vi "Test Program Read Tag Data.vi"(8 "error in (no error)":errorcluster, 10 "Data Cluster":T1, 11 "Task D-O Channels":string[][](array[string])) -> (0 "error out":errorcluster, 3 "Array":bool[][](array[boolean]))   [LabVIEW 2018, in "DAQ.lvlib"]
uses:
  DAQ.lvlib
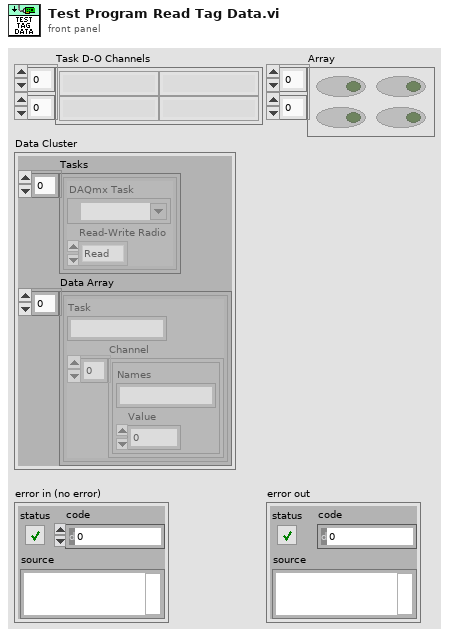
[diagram p1: front panel]
types:
  T1 = cluster{"Tasks":cluster{"DAQmx Task":refnum<k21>, "Read-Write Radio":enum32{"Read", "Write"}}[], "Data Array":cluster{"Task":string, "Channel":cluster{"Names":string, "Value":dbl}[]}[]}
  T2 = cluster{"Task":string, "Channel":cluster{"Names":string, "Value":dbl}[]}[]
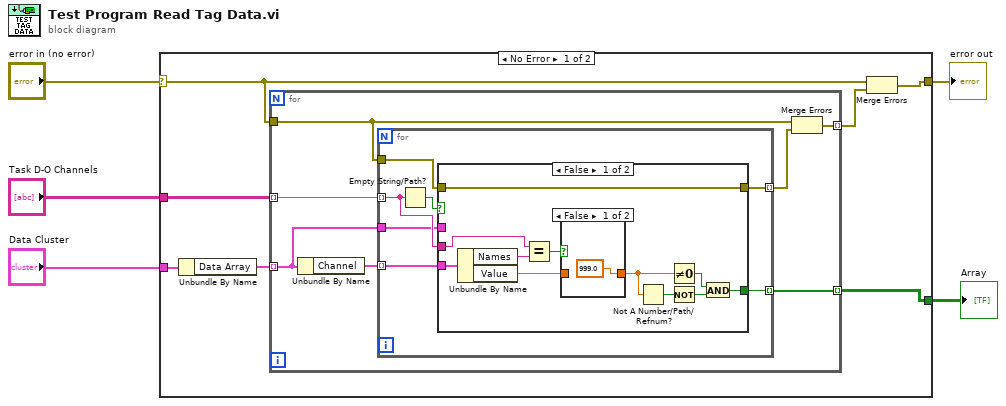
[diagram p0: block diagram]
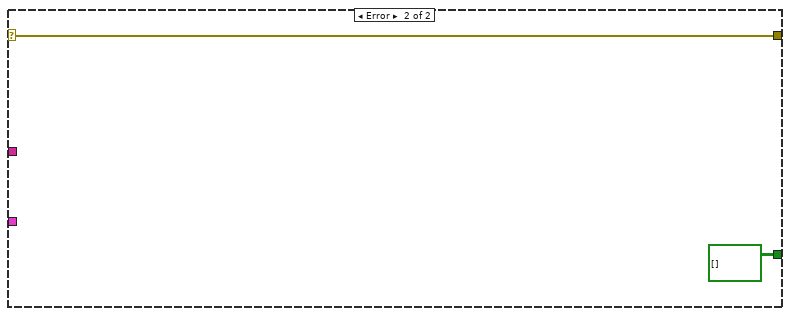
[diagram p4: hidden frame]
diagram:
  n1 = case shown="No Error" "error in (no error)" {
    selector: "error in (no error)" -> [w9 w42]
    tunnel: [w8 w42] -> w5
    tunnel: "Task D-O Channels" -> [w12 _]
    tunnel: [w11 bool[][] []] -> w3
    tunnel: "Data Cluster" -> [w7 _]
    frame No Error {
      n2 = Unbundle By Name(w7) -> ("Data Array"=w6:T2)
      n3 = for {
        tunnel: [w19] -> w10 mode=indexing
        tunnel: w12 -> [w16] mode=indexing
        tunnel: w9 -> [w15]
        tunnel: [w17] -> w11 mode=indexing
        tunnel: w6 -> [w14] mode=indexing
        n4 = Unbundle By Name(w14) -> ("Channel"=w13:cluster{"Names":string, "Value":dbl}[])
        n5 = for {
          tunnel: [w24] -> w17 mode=indexing
          tunnel: w16 -> [w22] mode=indexing
          tunnel: w15 -> [w26]
          tunnel: [w25] -> w18 mode=indexing
          tunnel: w14 -> [w21]
          tunnel: w13 -> [w20] mode=indexing
          n6 = Empty String/Path?(string/path=w22) -> (empty?=w23:bool)
          n7 = case shown="False" w23 {
            tunnel: w22 -> [w31 _]
            tunnel: w26 -> [w27 w40]
            tunnel: [w27 w40] -> w25
            tunnel: [w36 _] -> w24
            tunnel: w21 -> [_ _]
            tunnel: w20 -> [w33 _]
            frame False {
              n8 = Unbundle By Name(w33) -> ("Names"=w32:string, "Value"=w29:dbl)
              n9 = Equal?(x=w31, y=w32) -> (x = y?=w30:bool)
              n10 = case shown="False" w30 {
                tunnel: [999.0 w39] -> w28
                tunnel: w29 -> [_ w39]
                frame False {
                }
                frame True {
                }
              }
              n11 = Not A Number/Path/Refnum?(number/path/refnum=w28) -> (NaN/Path/Refnum?=w35:bool)
              n12 = Not Equal To 0?(x=w28) -> (x != 0?=w37:bool)
              n13 = Not(x=w35) -> (.not. x?=w34:bool)
              n14 = And(x=w37, y=w34) -> (x .and. y?=w36:bool)
            }
            frame True {
            }
          }
        }
        n15 = Merge Errors(w15, w18) -> (w19:errorcluster)
      }
      n16 = Merge Errors(w9, w10) -> (w8:errorcluster)
    }
    frame Error {
    }
  }
  "error out" <- w5
  "Array" <- w3
